vi "FTW-FileSystem-PathToURI.vi"(0 "Path":path, 11 "error in":errorcluster) -> (4 "URI":string, 15 "error out":errorcluster)   [LabVIEW 2012]
panel:
  # "Inputs"
  # "Outputs"
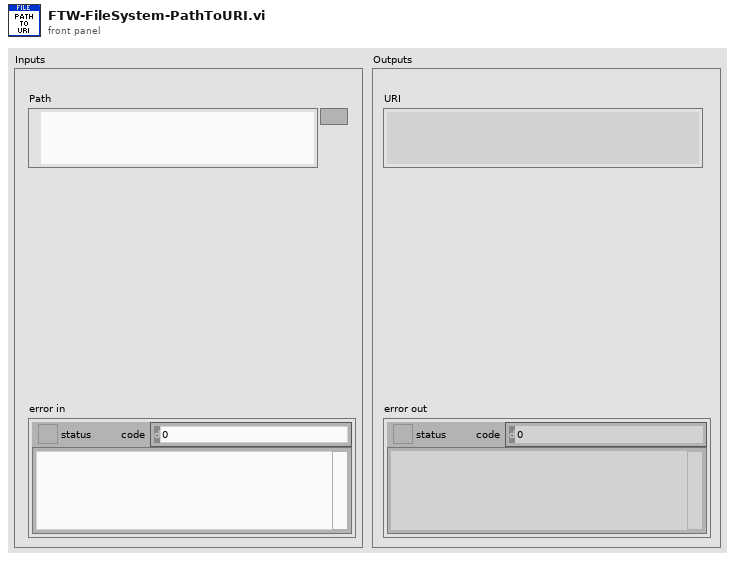
[diagram p1: front panel]
types:
  T1 = enum32{"invalid OS target", "Mac OS", "Windows 3.1", "Windows 95/NT", "Solaris 1", "Solaris 2", "HP-UX", "PowerMAX", "Linux", "Irix", "Rhapsody", "BeOS", "AIX", "OSF1", "VxWorks", "PharLap", "Carbon", "RTX", "Windows x64", "Linux x64"}
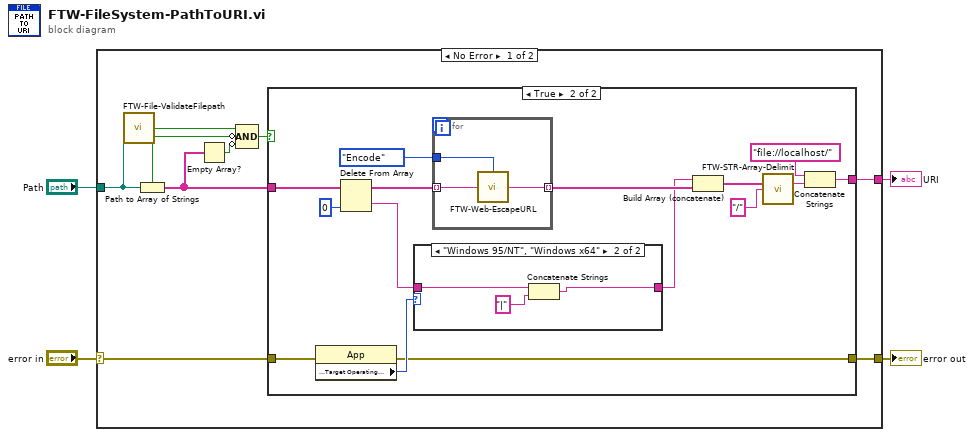
[diagram p0: block diagram]
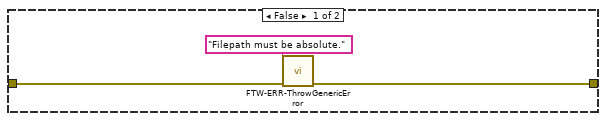
[diagram p2: hidden frame]
diagram:
  n1 = case shown="No Error" "error in" {
    selector: "error in" -> [w7 w39]
    tunnel: [w9 _] -> w4
    tunnel: "Path" -> [w8 _]
    tunnel: [w6 w39] -> w1
    frame No Error {
      n2 = call "FTW-File-ValidateFilepath.vi"("Filepath"=w8) -> ("Valid?"=w10:bool)
      n3 = Path to Array of Strings(0:w8) -> (1:w11:bool, 2:w13:string[])
      n4 = Empty Array?(array=w13) -> (empty?=w12:bool)
      n5 = Compound Arithmetic op=AND(w10, invert w11, invert w12) -> (w5:bool)
      n6 = case shown="True" w5 {
        tunnel: w13 -> [_ w24]
        tunnel: [_ w20] -> w9
        tunnel: w7 -> [w16 w19]
        tunnel: [w15 w18] -> w6
        frame False {
          n7 = call "FTW-ERR-ThrowGenericError.vi"("Error Message"="Filepath must be absolute.", "error in"=w16) -> ("error out"=w15:errorcluster)  [unwired: 13 in]
        }
        frame True {
          n8 = property class="App"(error in=w19) -> (error out=w18:errorcluster, "Application:Target Operating System"=w27:T1)  [unwired: 1 in, 1 out]
          n9 = Delete From Array(array=w24, index=0) -> (deleted portion=w28:string, array with subset deleted=w25:string[])  [unwired: 1 in]
          n10 = case shown="\"Windows 95/NT\", \"Windows x64\"" w27 {
            tunnel: w28 -> [w32 w35]
            tunnel: [w32 w33] -> w29
            frame Default {
            }
            frame "Windows 95/NT", "Windows x64" {
              n11 = Concatenate Strings(w35, "|" ("string")) -> (w33:string)
            }
          }
          n12 = for {
            tunnel: w25 -> [w38] mode=indexing
            tunnel: [w37] -> w31 mode=indexing
            tunnel: enum16{"Encode", "Decode"}."Encode" ("Direction") -> [w36]
            n13 = call "FTW-Web-EscapeURL.vi"("Input"=w38, "Direction"=w36) -> ("Output"=w37:string)
          }
          n14 = Build Array (concatenate)(w29, w31) -> (w30:string[])
          n15 = call "FTW-STR-Array-Delimit.vi"("Array of Strings"=w30, "Delimiter"="/") -> ("Delimited String"=w23:string)  [unwired: 13 in]
          n16 = Concatenate Strings("file://localhost/", w23) -> (w20:string)
        }
      }
    }
    frame Error {
    }
  }
  "error out" <- w1
  "URI" <- w4
